vi "RT Main.vi"   [LabVIEW 2020]
doc: "This template is for the Queued Message Handler design pattern.\n\nThe Event Handling Loop generates messages based on user interface actions.\n\nThe Message Handling Loop processes messages generated by the Event Handling Loop, or by other messages. The messages are string values, so new messages can be added easily to the Message Cases case structure in the Message Handling Loop. Each message cluster can also provide an optional value for Message Data, which is a variant that can be converted to whatever message-specific data is required."
uses:
  support/Message Queue/Message Queue.lvlib
  Globals/Global - All RT Loop Stop.vi
  controls/Raw Values.ctl
  <vilib>/rvi/interface/nirviReadWriteControl/nirviReadWriteControl.xnode
  controls/FPGA VI Reference.ctl
  <vilib>/rvi/errors/niLvFpgaAdjustHostInterfaceError.vi
  controls/Control Configuration.ctl
  controls/FPGA State.ctl
  Globals/Global - Configuration Options.vi
  <vilib>/rvi/interface/nirviCloseFPGA/nirviCloseFPGA.xnode
  Globals/Global - RT Stream Connections.vi
  NiFpgaLv.dll
  <vilib>/rvi/interface/Simulation/niFpgaSimulationCallBeginRW.vi
  <vilib>/nisyscfg/nisyscfg.lvlib
  <vilib>/FPGAPlugInAG/Dynamic/niLvFpga_Close_Dynamic.vi
types:
  T1 = typedef "FPGA VI Reference.ctl" = refnum<k20>
  T2 = typedef "FPGA State.ctl" = enum16{"Safe State", "Manual", "Control (PID)"}
  T3 = typedef "Raw Values.ctl" = cluster{"Channel 0":fxp<+/-,20,5>, "Channel 1":fxp<+/-,20,5>, "Channel 2":fxp<+/-,20,5>, "Channel 3":fxp<+/-,20,5>}
  T4 = typedef "Control Configuration.ctl" = cluster{"PID Gains":cluster{"proportional gain (Kc)":fxp<+/-,16,8>, "integral gain (Kc*Ts/Ti)":fxp<+/-,16,8>, "derivative gain (Kc*Td/Ts)":fxp<+/-,16,8>}, "Output Range":cluster{"output high":fxp<+/-,16,5>, "output low":fxp<+/-,16,5>}}
  T5 = typedef "All FPGA Configuration Values.ctl" = cluster{"FPGA State":T2, "Manual Values":T3, "Setpoints":T3, "Control Configurations":T4[]}
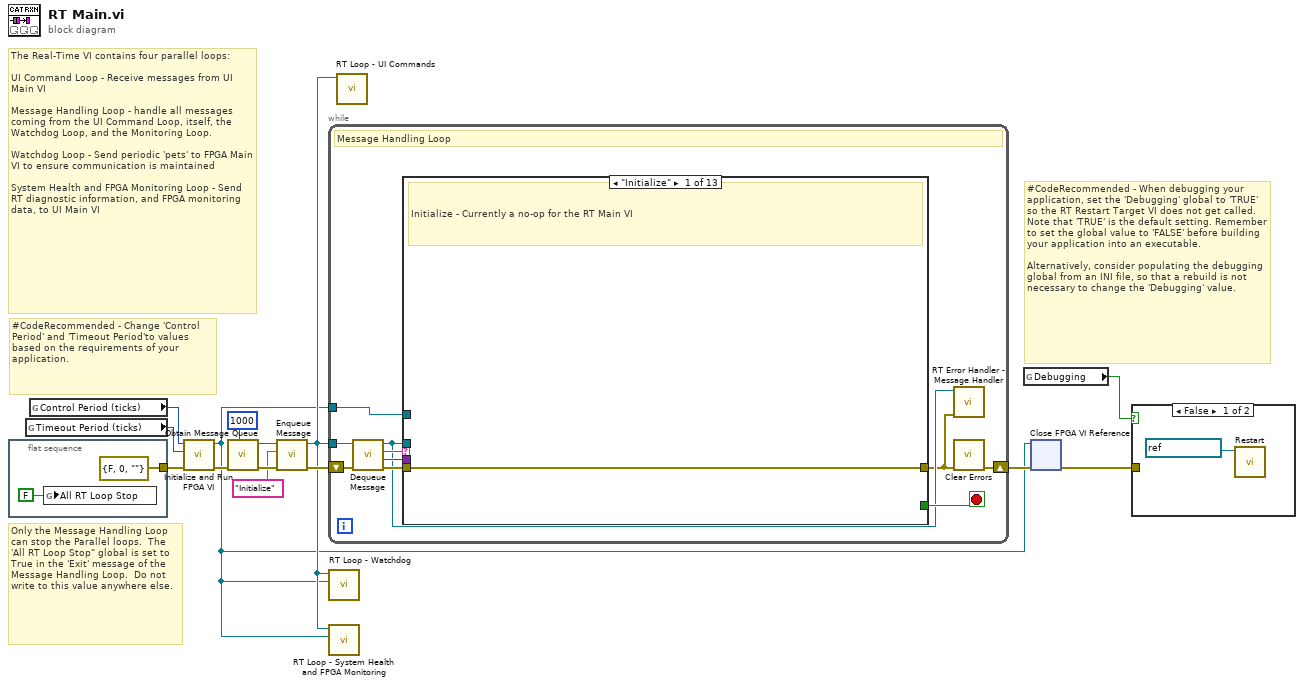
[diagram p0: block diagram]
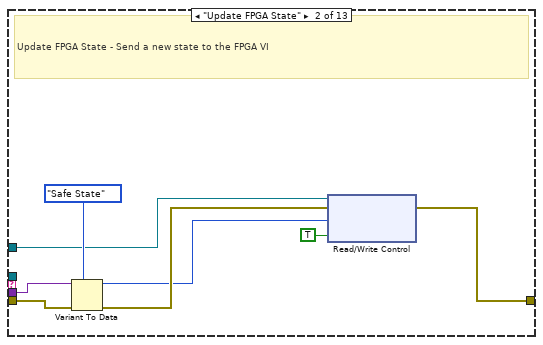
[diagram p3: hidden frame]
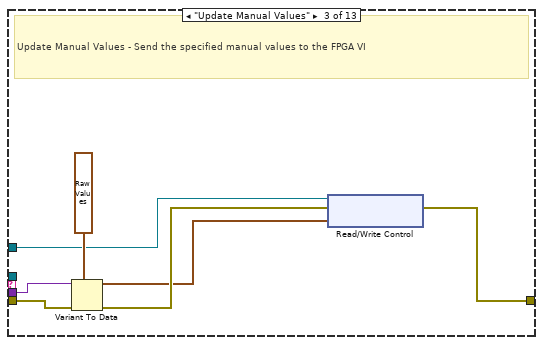
[diagram p4: hidden frame]
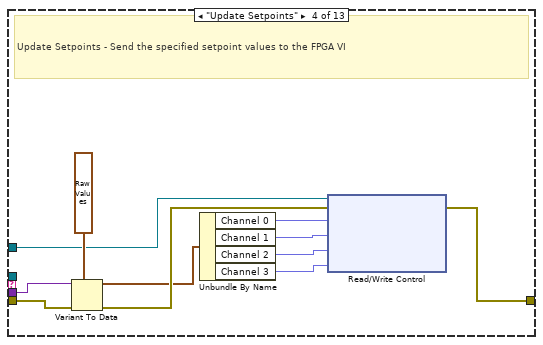
[diagram p5: hidden frame]
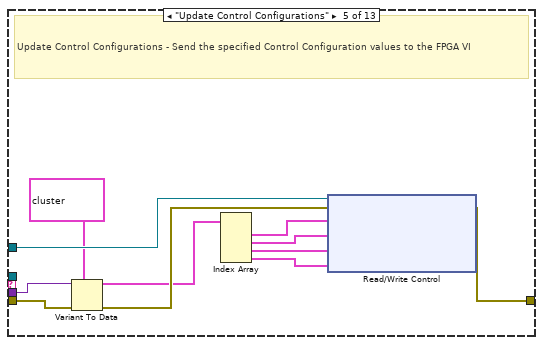
[diagram p6: hidden frame]
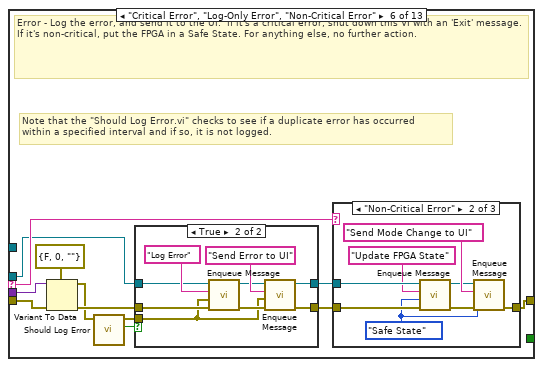
[diagram p7: hidden frame]
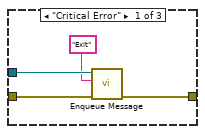
[diagram p9: hidden frame]
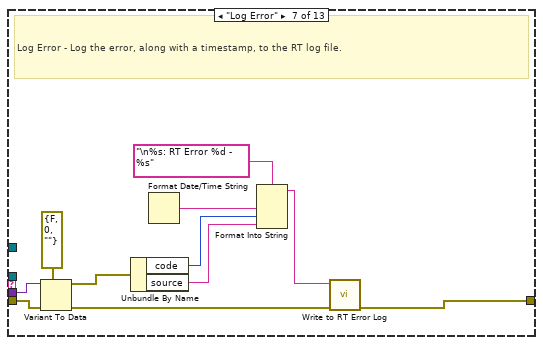
[diagram p11: hidden frame]
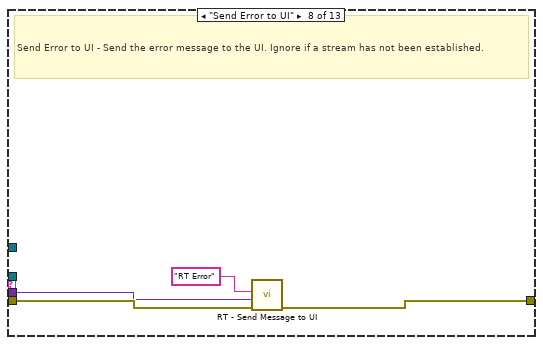
[diagram p12: hidden frame]
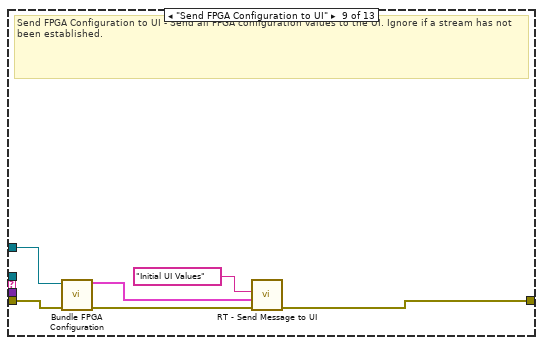
[diagram p13: hidden frame]
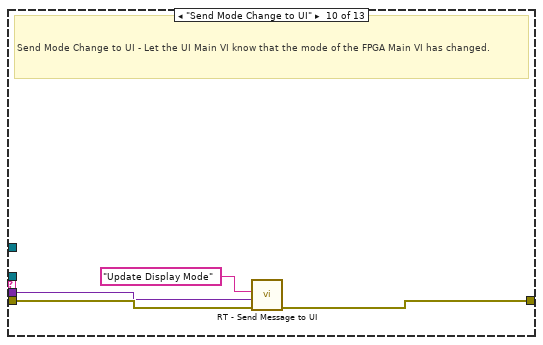
[diagram p14: hidden frame]
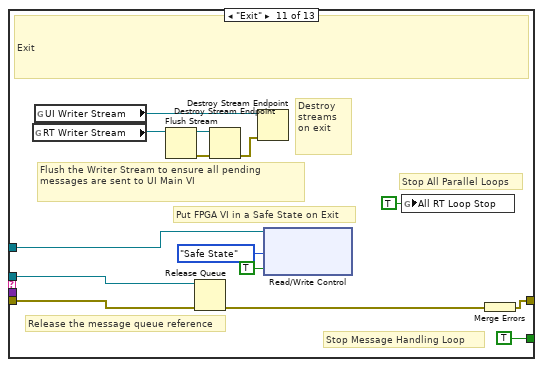
[diagram p15: hidden frame]
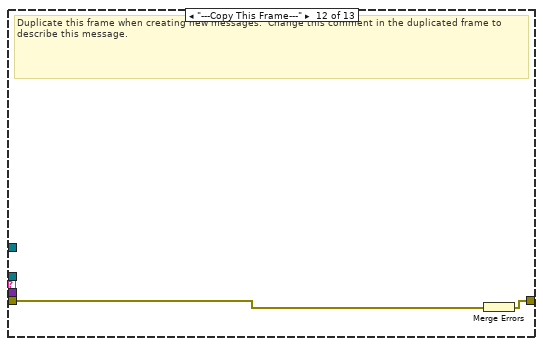
[diagram p16: hidden frame]
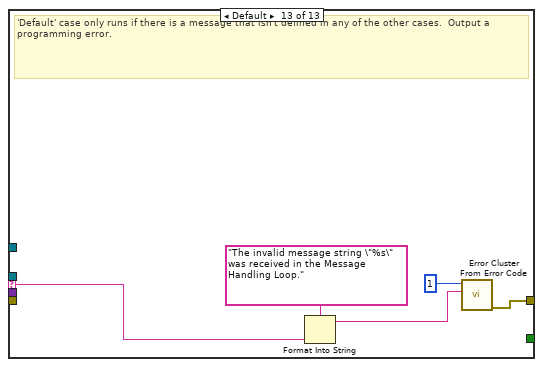
[diagram p17: hidden frame]
diagram:
  # "#CodeRecommended - When debugging your application, set the 'Debugging' global to 'TRUE' so the RT Restart Target VI does not get called.  Note that 'TRUE' is the default setting. Remember to set the global value to 'FALSE' before building your application into an executable.\n\nAlternatively, consider populating the debugging global from an INI file, so that a rebuild is not necessary to change the 'Debugging' value."
  # "#CodeRecommended - Change 'Control Period' and 'Timeout Period'to values based on the requirements of your application."
  # "The Real-Time VI contains four parallel loops:\n\nUI Command Loop - Receive messages from UI Main VI\n\nMessage Handling Loop - handle all messages coming from the UI Command Loop, itself, the Watchdog Loop, and the Monitoring Loop.\n\nWatchdog Loop - Send periodic 'pets' to FPGA Main VI to ensure communication is maintained\n\nSystem Health and FPGA Monitoring Loop - Send RT diagnostic information, and FPGA monitoring data, to UI Main VI"
  # "Only the Message Handling Loop can stop the Parallel loops.  The 'All RT Loop Stop\" global is set to True in the 'Exit' message of the Message Handling Loop.  Do not write to this value anywhere else."
  n1 = flat-sequence {
    tunnel: [errorcluster {"status"=FALSE, "code"=0, "source"=""} ("error constant")] -> w9
    frame #0 {
      n2 = global write "Global - All RT Loop Stop.vi" "All RT Loop Stop"(FALSE) -> ()
    }
  }
  n3 = global read "Global - Configuration Options.vi" "Timeout Period (ticks)"() -> (w7:u64)
  n4 = global read "Global - Configuration Options.vi" "Control Period (ticks)"() -> (w6:u32)
  n5 = call "Initialize and Run FPGA VI.vi"("error in (no error)"=w9, "Timeout Period (ticks)"=w7, "Control Period (ticks)"=w6) -> ("error out"=w10:errorcluster, "FPGA VI Reference Out"=w4:T1)  [unwired: 7 in]
  n6 = call "Obtain Message Queue.vi"("max queue size (-1, unlimited)"=1000, "error in (no error)"=w10) -> ("error out"=w14:errorcluster, "Message Queue"=w13:refnum<queue>)  [unwired: 8 in]
  n7 = call "Enqueue Message.vi"("error in (no error)"=w14, "Message"="Initialize", "Message Queue"=w13) -> ("error out"=w11:errorcluster, "dup Message Queue"=w8:refnum<queue>)  [unwired: 7 in]
  n8 = while {
    tunnel: w8 -> [w21]
    shift-right: [w18] -> w5
    shift-left: w11 -> [w25]
    tunnel: w4 -> [w20]
    stop <- w26 stop-if-true
    # "Message Handling Loop"
    n9 = call "Dequeue Message.vi"("error in (no error)"=w25, "Message Queue"=w21) -> ("error out"=w24:errorcluster, "Message Data"=w22:variant, "Message"=w23:string, "dup Message Queue"=w19:refnum<queue>)  [unwired: 6 in]
    n10 = case "Message Cases" shown="\"Initialize\"" w23 {
      selector: w23 -> [_ _ _ _ _ w74 _ _ _ _ _ _ w145]
      tunnel: w19 -> [_ _ _ _ _ w68 _ _ _ _ w139 _ _]
      tunnel: w24 -> [w27 w35 w42 w53 w64 w72 w111 w115 w121 w125 w135 w141 _]
      tunnel: [w27 w32 w39 w50 w62 w73 w102 w112 w116 w124 w136 w140 w143] -> w17
      tunnel: [_ _ _ _ _ _ _ _ _ _ TRUE _ _] -> w26
      tunnel: w22 -> [_ w34 w41 w52 w63 w71 w110 w114 _ w123 _ _ _]
      tunnel: w20 -> [_ w30 w37 w48 w60 _ _ _ w120 _ w131 _ _]
      frame "Initialize" {
        # "Initialize - Currently a no-op for the RT Main VI"
      }
      frame "Update FPGA State" {
        # "Update FPGA State - Send a new state to the FPGA VI"
        n11 = Variant To Data(error in=w35, type=FPGA_State."Safe State" ("FPGA State"), Variant=w34) -> (data=w29:T2, error out=w31:errorcluster)
        n12 = xnode "Read/Write Control"("FPGA VI Reference In"=w30, "error in"=w31, "New State"=w29, "Change State"=TRUE) -> ("error out"=w32:errorcluster)  [unwired: 1 out]
      }
      frame "Update Manual Values" {
        # "Update Manual Values - Send the specified manual values to the FPGA VI"
        n13 = Variant To Data(error in=w42, type=T3 {"Channel 0"=0.0, "Channel 1"=0.0, "Channel 2"=0.0, "Channel 3"=0.0} ("Raw Values"), Variant=w41) -> (data=w36:T3, error out=w38:errorcluster)
        n14 = xnode "Read/Write Control"("FPGA VI Reference In"=w37, "error in"=w38, "Manual Values"=w36) -> ("error out"=w39:errorcluster)  [unwired: 1 out]
      }
      frame "Update Setpoints" {
        # "Update Setpoints - Send the specified setpoint values to the FPGA VI"
        n15 = Variant To Data(error in=w53, type=T3 {"Channel 0"=0.0, "Channel 1"=0.0, "Channel 2"=0.0, "Channel 3"=0.0} ("Raw Values"), Variant=w52) -> (data=w47:T3, error out=w49:errorcluster)
        n16 = Unbundle By Name(w47) -> ("Channel 0"=w46:fxp<+/-,20,5>, "Channel 1"=w45:fxp<+/-,20,5>, "Channel 2"=w44:fxp<+/-,20,5>, "Channel 3"=w43:fxp<+/-,20,5>)
        n17 = xnode "Read/Write Control"("FPGA VI Reference In"=w48, "error in"=w49, "Channel 0 Setpoint"=w46, "Channel 1 Setpoint"=w45, "Channel 2 Setpoint"=w44, "Channel 3 Setpoint"=w43) -> ("error out"=w50:errorcluster)  [unwired: 1 out]
      }
      frame "Update Control Configurations" {
        # "Update Control Configurations - Send the specified Control Configuration values to the FPGA VI"
        n18 = Variant To Data(error in=w64, type=T4[] [{"PID Gains"={"proportional gain (Kc)"=0.0, "integral gain (Kc*Ts/Ti)"=0.0, "derivative gain (Kc*Td/Ts)"=0.0}, "Output Range"={"output high"=0.0, "output low"=0.0}}], Variant=w63) -> (data=w58:T4[], error out=w61:errorcluster)
        n19 = Index Array(array=w58) -> (element #1=w57:T4, element #2=w56:T4, element #3=w55:T4, element #4=w54:T4)  [unwired: 4 in]
        n20 = xnode "Read/Write Control"("FPGA VI Reference In"=w60, "error in"=w61, "Channel 0 Configuration"=w57, "Channel 1 Configuration"=w56, "Channel 2 Configuration"=w55, "Channel 3 Configuration"=w54) -> ("error out"=w62:errorcluster)  [unwired: 1 out]
      }
      frame "Critical Error", "Log-Only Error", "Non-Critical Error" {
        # "Note that the \"Should Log Error.vi\" checks to see if a duplicate error has occurred \nwithin a specified interval and if so, it is not logged."
        # "Error - Log the error, and send it to the UI.  If it's a critical error, shut down this VI with an 'Exit' message. If it's non-critical, put the FPGA in a Safe State. For anything else, no further action."
        n21 = Variant To Data(error in=w72, type=errorcluster {"status"=FALSE, "code"=0, "source"=""} ("error out"), Variant=w71) -> (data=w66:errorcluster, error out=w69:errorcluster)
        n22 = call "Should Log Error.vi"("error to report"=w66) -> ("Should Log Error?"=w67:bool, "dup error to report"=w65:errorcluster)  [unwired: 9 in]
        n23 = case shown="True" w67 {
          tunnel: [w78 w85] -> w76
          tunnel: [w77 w84] -> w75
          tunnel: w68 -> [w77 w83]
          tunnel: w69 -> [w78 w80]
          tunnel: w65 -> [_ w79]
          frame False {
          }
          frame True {
            n24 = call "Enqueue Message.vi"("error in (no error)"=w80, "Message Data"=w79, "Message"="Log Error", "Message Queue"=w83) -> ("error out"=w81:errorcluster, "dup Message Queue"=w82:refnum<queue>)  [unwired: 6 in]
            n25 = call "Enqueue Message.vi"("error in (no error)"=w81, "Message Data"=w79, "Message"="Send Error to UI", "Message Queue"=w82) -> ("error out"=w85:errorcluster, "dup Message Queue"=w84:refnum<queue>)  [unwired: 6 in]
          }
        }
        n26 = case shown="\"Non-Critical Error\"" w74 {
          tunnel: w76 -> [w91 w99 w100]
          tunnel: w75 -> [w89 w98 _]
          tunnel: [w90 w95 w100] -> w73
          frame "Critical Error" {
            n27 = call "Enqueue Message.vi"("error in (no error)"=w91, "Message"="Exit", "Message Queue"=w89) -> ("error out"=w90:errorcluster)  [unwired: 7 in, 1 out]
          }
          frame "Non-Critical Error" {
            w92 = FPGA_State."Safe State" ("FPGA State")
            n28 = call "Enqueue Message.vi"("error in (no error)"=w99, "Message Data"=w92, "Message"="Update FPGA State", "Message Queue"=w98) -> ("error out"=w96:errorcluster, "dup Message Queue"=w93:refnum<queue>)  [unwired: 6 in]
            n29 = call "Enqueue Message.vi"("error in (no error)"=w96, "Message Data"=w92, "Message"="Send Mode Change to UI", "Message Queue"=w93) -> ("error out"=w95:errorcluster)  [unwired: 6 in, 1 out]
          }
          frame Default {
          }
        }
      }
      frame "Log Error" {
        # "Log Error - Log the error, along with a timestamp, to the RT log file."
        n30 = Variant To Data(error in=w111, type=errorcluster {"status"=FALSE, "code"=0, "source"=""} ("error constant"), Variant=w110) -> (data=w105:errorcluster, error out=w108:errorcluster)
        n31 = Unbundle By Name(w105) -> ("code"=w104:i32, "source"=w103:string)
        n32 = Format Date/Time String() -> (date/time string=w106:string)  [unwired: 3 in]
        n33 = Format Into String(format string="\n%s: RT Error %d - %s", w106, w104, w103) -> (resulting string=w101:string)  [unwired: 2 in, 1 out]
        n34 = call "Write to RT Error Log.vi"("error in (no error)"=w108, "Log Entry"=w101) -> ("error out"=w102:errorcluster)  [unwired: 9 in]
      }
      frame "Send Error to UI" {
        # "Send Error to UI - Send the error message to the UI. Ignore if a stream has not been established."
        n35 = call "RT - Send Message to UI.vi"("error in (no error)"=w115, "Message Data"=w114, "Message"="RT Error") -> ("error out"=w112:errorcluster)  [unwired: 8 in]
      }
      frame "Send FPGA Configuration to UI" {
        # "Send FPGA Configuration to UI - Send all FPGA configuration values to the UI. Ignore if a stream has not been established."
        n36 = call "Bundle FPGA Configuration.vi"("error in (no error)"=w121, "FPGA Interface"=w120) -> ("error out"=w119:errorcluster, "All FPGA Configuration Values"=w118:T5)  [unwired: 8 in]
        n37 = call "RT - Send Message to UI.vi"("error in (no error)"=w119, "Message Data"=w118, "Message"="Initial UI Values") -> ("error out"=w116:errorcluster)  [unwired: 8 in]
      }
      frame "Send Mode Change to UI" {
        # "Send Mode Change to UI - Let the UI Main VI know that the mode of the FPGA Main VI has changed."
        n38 = call "RT - Send Message to UI.vi"("error in (no error)"=w125, "Message Data"=w123, "Message"="Update Display Mode") -> ("error out"=w124:errorcluster)  [unwired: 8 in]
      }
      frame "Exit" {
        # "Flush the Writer Stream to ensure all pending messages are sent to UI Main VI"
        # "Destroy streams on exit"
        # "Put FPGA VI in a Safe State on Exit"
        # "Stop Message Handling Loop"
        # "Stop All Parallel Loops"
        # "Release the message queue reference"
        # "Exit"
        n39 = global read "Global - RT Stream Connections.vi" "RT Writer Stream"() -> (w128:refnum<k21>)
        n40 = global read "Global - RT Stream Connections.vi" "UI Writer Stream"() -> (w130:refnum<k21>)
        n41 = Flush Stream(11:w128) -> (0:w126:errorcluster, 3:w127:refnum<k21>)  [unwired: 3 in, 1 out]
        n42 = Release Queue(queue=w139, error in (no error)=w135) -> (error out=w137:errorcluster)  [unwired: 1 in, 2 out]
        n43 = Destroy Stream Endpoint(8:w126, 11:w127) -> (0:w129:errorcluster)
        n44 = Destroy Stream Endpoint(8:w129, 11:w130) -> ()  [unwired: 1 out]
        n45 = xnode "Read/Write Control"("FPGA VI Reference In"=w131, "New State"=FPGA_State."Safe State", "Change State"=TRUE) -> ()  [unwired: 1 in, 2 out]
        n46 = global write "Global - All RT Loop Stop.vi" "All RT Loop Stop"(TRUE ("Stop Monitoring Loops")) -> ()
        n47 = Merge Errors(w137) -> (w136:errorcluster)
      }
      frame "---Copy This Frame---" {
        # "Duplicate this frame when creating new messages.  Change this comment in the duplicated frame to describe this message."
        n48 = Merge Errors(w141) -> (w140:errorcluster)
      }
      frame Default {
        # "'Default' case only runs if there is a message that isn't defined in any of the other cases.  Output a programming error."
        n49 = Format Into String(format string="The invalid message string \"%s\" was received in the Message Handling Loop." ("Unknown Message Error Text"), w145) -> (resulting string=w142:string)  [unwired: 2 in, 1 out]
        n50 = call <vilib>:"Error Cluster From Error Code.vi"("error message (\"\")"=w142, "error code (0)"=1) -> ("error out"=w143:errorcluster)  [unwired: 7 in]
      }
    }
    n51 = call "RT Error Handler - Message Handler.vi"("error in (no error)"=w17, "Message Queue"=w19) -> ()  [unwired: 9 in, 1 out]
    n52 = call <vilib>:"Clear Errors.vi"("error in (no error)"=w17) -> ("error out"=w18:errorcluster)  [unwired: 5 in, 1 out]
  }
  n53 = call "RT Loop - Watchdog.vi"("FPGA VI Reference"=w4, "Message Queue"=w8) -> ()  [unwired: 10 in]
  n54 = call "RT Loop - System Health and FPGA Monitoring.vi"("FPGA VI Reference"=w4, "Message Queue"=w8) -> ()  [unwired: 10 in]
  n55 = call "RT Loop - UI Commands.vi"("Message Queue"=w8) -> ()  [unwired: 11 in]
  n56 = global read "Global - Configuration Options.vi" "Debugging"() -> (w2:bool)
  n57 = xnode "Close FPGA VI Reference"("FPGA VI Reference In"=w4, "error in"=w5) -> ("error out"=w3:errorcluster)
  n58 = case shown="False" w2 {
    tunnel: w3 -> [_ _]
    frame False {
      n59 = call <vilib>:"Restart.vi"("Session in"=refnum<k21> "localhost" ("session in")) -> ()  [unwired: 8 in, 3 out]
    }
    frame True {
    }
  }
